vi "Transfer Configuration.Initialize.vi"(7 "direction":T1, 8 "error in (no error)":errorcluster, 10 "Transfer Configuration cluster":T2, 11 "Transfer Configuration in":refnum<class "Transfer Configuration.lvclass">) -> (0 "error out":errorcluster, 3 "Transfer Configuration out":refnum<class "Transfer Configuration.lvclass">)   [LabVIEW 2017, in "DSF.Engine.lvlib" / "Transfer Configuration.lvclass"]
uses:
  Transfer Configuration.lvclass
  C:/Git/DSF/DSF Core/Source/Shared/Classes/Configuration/Configuration.lvclass
  DSF Configuration API/1.0.0/Public/Controls/DSF Engine Transfer Configuration.ctl
  DSF Configuration API/1.0.0/Public/Controls/DSF Byte Order.ctl
  DSF Configuration API/1.0.0/Public/Controls/DSF Engine Channel Configuration.ctl
  DSF Configuration API/1.0.0/Public/Controls/DSF Data Type.ctl
  DSF Configuration API/1.0.0/Public/Controls/DSF Settings Info.ctl
  DSF Configuration API/1.0.0/Public/Controls/DSF Direction.ctl
  Configuration/Configuration.lvclass/Configuration.ctl
  Transfer Configuration.lvclass/Transfer Configuration.ctl
  Typedefs/DSF Runtime Channel Block.ctl
  DSF.Engine.lvlib
  DSF Configuration API/1.0.0/DSF Configuration API.lvlib
  Configuration/Configuration.lvclass
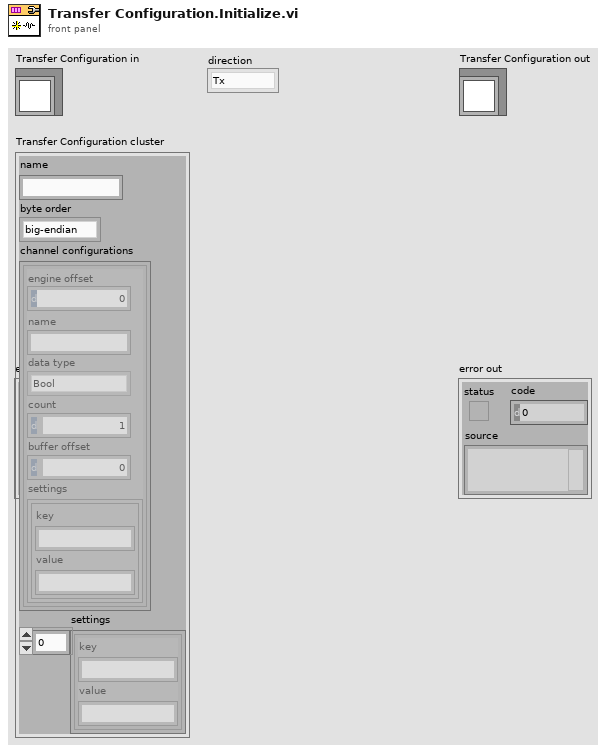
[diagram p1: front panel]
types:
  T1 = typedef "DSF Configuration API.lvlib/DSF Direction.ctl" = enum8{"Tx", "Rx"}
  T2 = typedef "DSF Configuration API.lvlib/DSF Engine Transfer Configuration.ctl" = cluster{"name":string, "byte order":T3, "channel configurations":T4[], "settings":T6}
  T3 = typedef "DSF Configuration API.lvlib/DSF Byte Order.ctl" = enum8{"big-endian", "little-endian"}
  T4 = typedef "DSF Configuration API.lvlib/DSF Engine Channel Configuration.ctl" = cluster{"engine offset":u64, "name":string, "data type":T5, "count":u64, "buffer offset":u64, "settings":T6}
  T5 = typedef "DSF Configuration API.lvlib/DSF Data Type.ctl" = enum8{"Bool", "SGL", "DBL", "I8", "I16", "I32", "I64", "U8", "U16", "U32", "U64"}
  T6 = typedef "DSF Configuration API.lvlib/DSF Settings Info.ctl" = cluster{"key":string, "value":string}[]
  T7 = typedef "DSF.Engine.lvlib/DSF Runtime Channel Block.ctl" = cluster{"data type":T5, "count":u64, "buffer offset":u64}
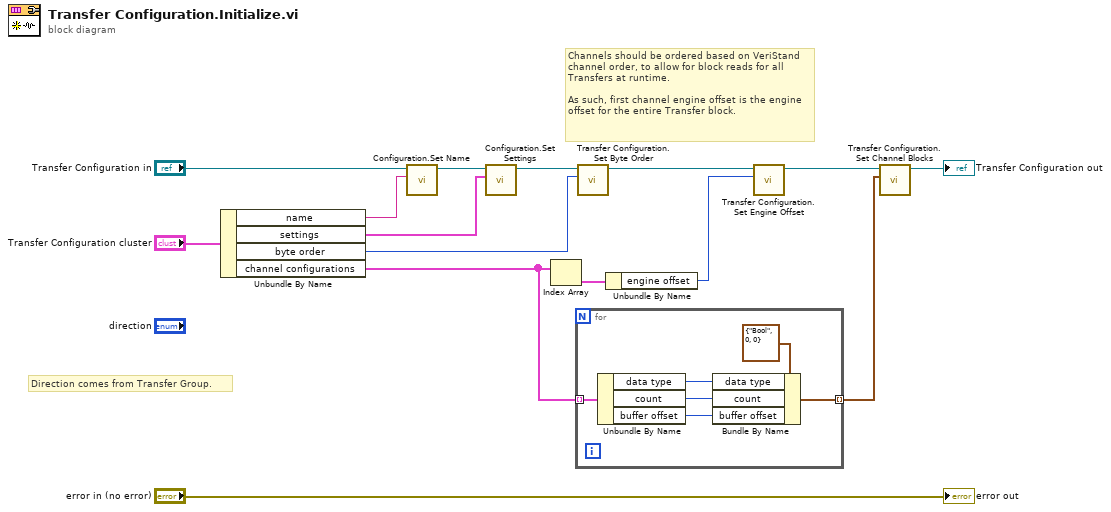
[diagram p0: block diagram]
diagram:
  # "Direction comes from Transfer Group."
  # "Channels should be ordered based on VeriStand channel order, to allow for block reads for all Transfers at runtime.\n\nAs such, first channel engine offset is the engine offset for the entire Transfer block."
  n1 = Unbundle By Name("Transfer Configuration cluster") -> ("name"=w6:string, "settings"=w2:T6, "byte order"=w7:T3, "channel configurations"=w12:T4[])
  n2 = call "Configuration.Set Name.vi"("name"=w6, "Configuration in"="Transfer Configuration in") -> ("Configuration out"=w4:refnum<class "Transfer Configuration.lvclass">)  [unwired: 9 in]
  n3 = call "Configuration.Set Settings.vi"("settings"=w2, "Configuration in"=w4) -> ("Configuration out"=w3:refnum<class "Transfer Configuration.lvclass">)  [unwired: 9 in]
  n4 = Index Array(array=w12) -> (element=w13:T4)  [unwired: 1 in]
  n5 = for {
    tunnel: w12 -> [w20] mode=indexing
    tunnel: [w16] -> w10 mode=indexing
    n6 = Unbundle By Name(w20) -> ("data type"=w19:T5, "count"=w18:u64, "buffer offset"=w17:u64)
    n7 = Bundle By Name(cluster=T7 {"data type"=enum."Bool", "count"=0, "buffer offset"=0} ("Channel Block"), "data type"=w19, "count"=w18, "buffer offset"=w17) -> (w16:T7)
  }
  n8 = call "Transfer Configuration.Set Byte Order.vi"("byte order"=w7, "Transfer Configuration in"=w3) -> ("Transfer Configuration out"=w8:refnum<class "Transfer Configuration.lvclass">)  [unwired: 9 in]
  n9 = Unbundle By Name(w13) -> ("engine offset"=w14:u64)
  n10 = call "Transfer Configuration.Set Engine Offset.vi"("engine offset"=w14, "Transfer Configuration in"=w8) -> ("Transfer Configuration out"=w1:refnum<class "Transfer Configuration.lvclass">)  [unwired: 9 in]
  n11 = call "Transfer Configuration.Set Channel Blocks.vi"("channel blocks"=w10, "Transfer Configuration in"=w1) -> ("Transfer Configuration out"=→"Transfer Configuration out":refnum<class "Transfer Configuration.lvclass">)  [unwired: 9 in]
  "error out" <- "error in (no error)"
